vi "Get Broadcast Event.vi"(8 "error in (no error)":errorcluster, 11 "Application in":refnum<class "Application.lvclass">) -> (0 "error out":errorcluster, 2 "Broadcast Event":refnum<user-event>[](array[refnum]), 3 "Application out":refnum<class "Application.lvclass">)   [LabVIEW 2020, in "Application.lvclass"]
doc: "Recursively get the broadcast event used to send broadcasts to registered observers."
uses:
  Application.lvclass
  Process/Protected/Broadcasting/Broadcast Message Cluster.ctl
  Process/Process.lvclass/Process.ctl
  Application.lvclass/Application.ctl
  Process/Public/Lifecycle/Get Lifecycle State.vi
  Process/Protected/Messaging/Request Message.vi
  <vilib>/Utility/error.llb/Clear Errors.vi
  Process/Private/SubVIs/Enqueue Request Message.vi
  <vilib>/AdvancedString/1D String Array to Delimited String.vi
  <vilib>/Utility/error.llb/Error Cluster From Error Code.vi
  Process/Private/SubVIs/Wait for Response Message.vi
  Process/Process.lvclass
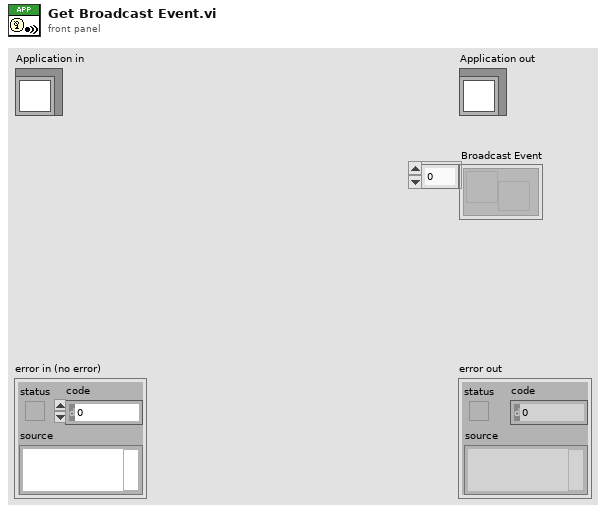
[diagram p1: front panel]
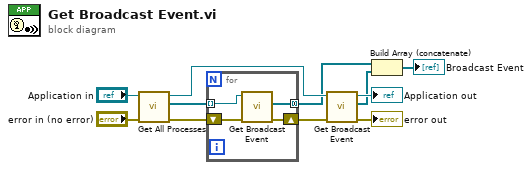
[diagram p0: block diagram]
diagram:
  n1 = call "Get All Processes.vi"("error in (no error)"="error in (no error)", "Application In"="Application in") -> ("error out"=w3:errorcluster, "App Processes"=w8:refnum<class "Process.lvclass">[], "Application Out"=w7:refnum<class "Application.lvclass">)  [unwired: 7 in]
  n2 = for {
    tunnel: w8 -> [w15] mode=indexing
    tunnel: [w12] -> w6 mode=concatenating
    shift-right: [w14] -> w4
    shift-left: w3 -> [w13]
    n3 = call-dynamic "Get Broadcast Event.vi"("error in (no error)"=w13, "Process in"=w15) -> ("error out"=w14:errorcluster, "Broadcast Event"=w12:refnum<user-event>[])  [unwired: 7 in, 1 out]
  }
  n4 = call-parent "Get Broadcast Event.vi"("error in (no error)"=w4, "Process in"=w7) -> ("error out"=→"error out":errorcluster, "Broadcast Event"=w5:refnum<user-event>[], "Process out"=→"Application out":refnum<class "Application.lvclass">)  [unwired: 7 in]
  n5 = Build Array (concatenate)(w6, w5) -> (→"Broadcast Event":refnum<user-event>[])
